vi "PXI-Set Auto Ramping.vi"(0 "Auto ramp?":bool, 7 "Ramp duration (ms)":dbl=5.0, 11 "error in (no error)":errorcluster) -> (15 "error out":errorcluster)   [LabVIEW 2020]
uses:
  Type Defs/Ramping Params.ctl
  DAQ Engine VIs/PXI Globals.vi
panel:
  in  "Ramping":T1={"Ramp up?"=FALSE, "Ramp down?"=FALSE, "Ramp duration (msecs)"=0.005, "Ramp type"=enum."Cos2"}
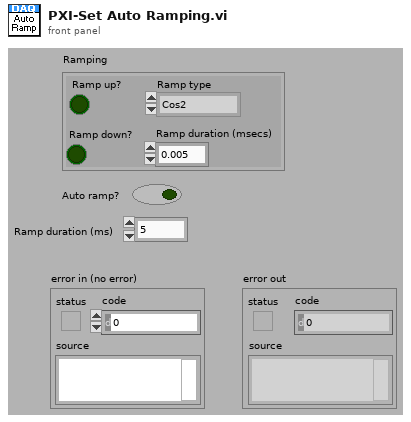
[diagram p1: front panel]
types:
  T1 = typedef "Ramping Params.ctl" = cluster{"Ramp up?":bool, "Ramp down?":bool, "Ramp duration (msecs)":dbl, "Ramp type":enum16{"Linear", "Cos2"}}
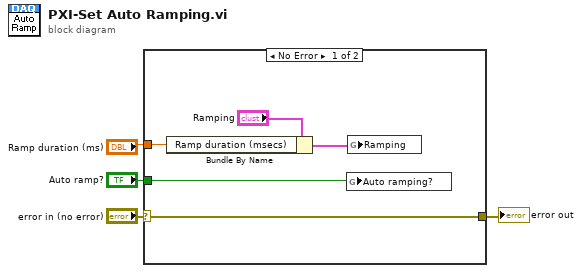
[diagram p0: block diagram]
diagram:
  n1 = case shown="No Error" "error in (no error)" {
    selector: "error in (no error)" -> [w6 w10]
    tunnel: "Auto ramp?" -> [w5 _]
    tunnel: "Ramp duration (ms)" -> [w8 _]
    tunnel: [w6 w10] -> w1
    frame No Error {
      n2 = Bundle By Name(cluster="Ramping", "Ramp duration (msecs)"=w8) -> (w7:T1)
      n3 = global write "PXI Globals.vi" "Auto ramping?"(w5) -> ()
      n4 = global write "PXI Globals.vi" "Ramping"(w7) -> ()
    }
    frame Error {
    }
  }
  "error out" <- w1
